vi "vizuXY_svi.vi"(9 "LY (mm)":dbl, 10 "LX (mm)":dbl, 11 "stored XY (µm)":T1 caption="stored XY") -> (3 "Tableau":T2(array[cluster]))   [LabVIEW 2013]
uses:
  <vilib>/Analysis/Matrix/Datatypes/RealMatrix.ctl
  <vilib>/Analysis/Matrix/Numeric/Conversions/Matrix To Array - RM.vi
  <vilib>/Analysis/Matrix/NI_Matrix.lvlib
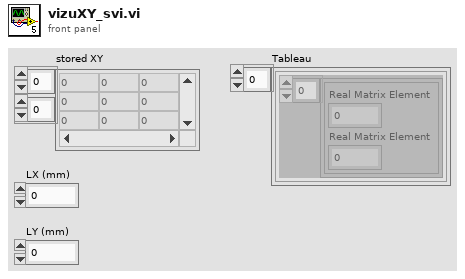
[diagram p1: front panel]
types:
  T1 = typedef "NI_Matrix.lvlib/RealMatrix.ctl" = dbl[][]
  T2 = cluster{cluster{"Real Matrix Element":dbl, "Real Matrix Element":dbl}[]}[]
  T3 = cluster{"Real Matrix Element":dbl, "Real Matrix Element":dbl}
  T4 = cluster{cluster{"Real Matrix Element":dbl, "Real Matrix Element":dbl}[]}
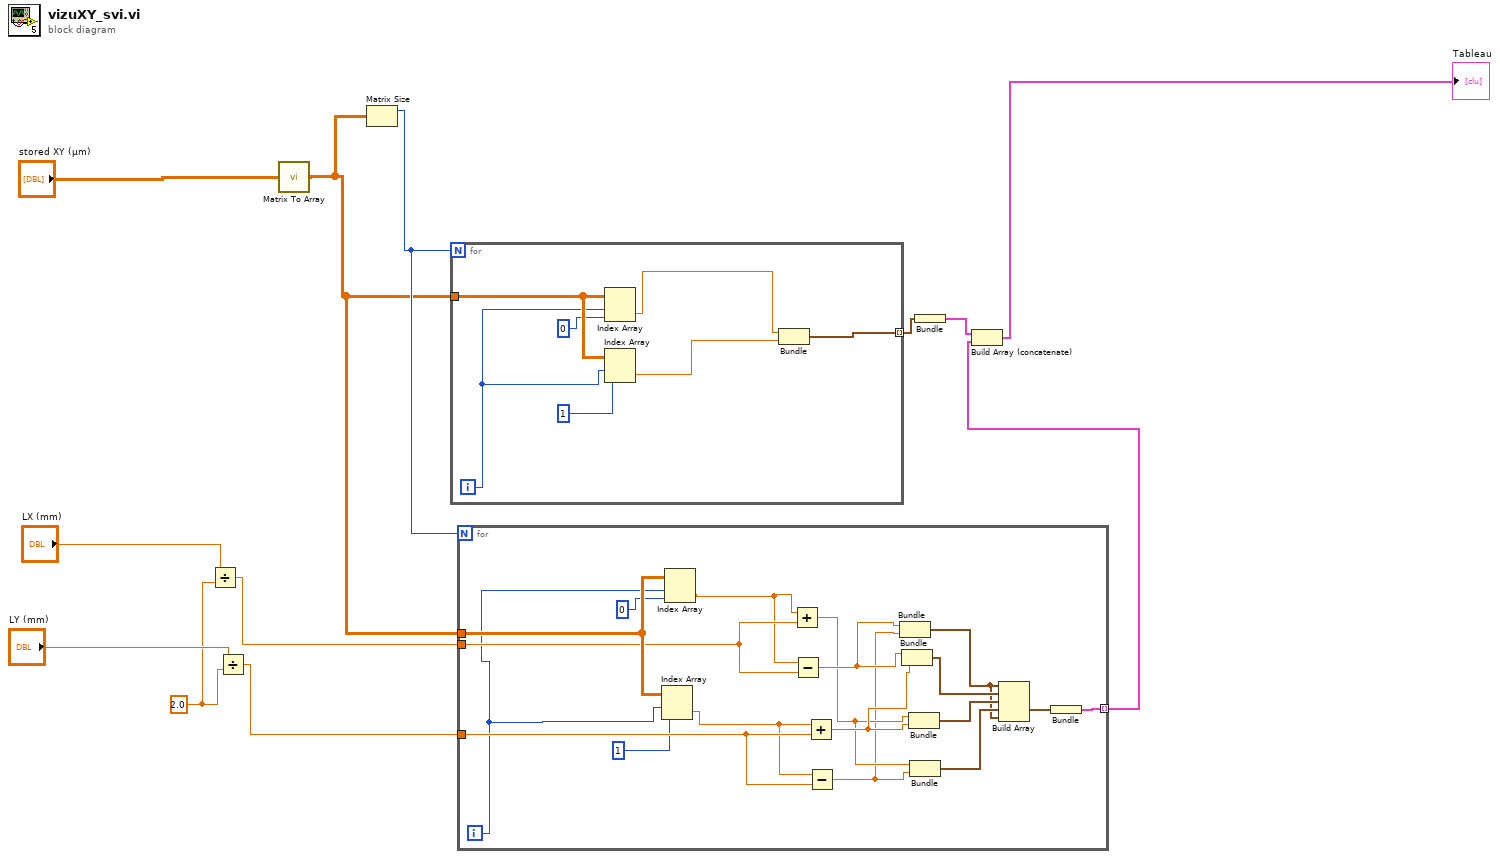
[diagram p0: block diagram]
diagram:
  w5 = 2.0
  n1 = Divide(x="LX (mm)", y=w5) -> (x/y=w6:dbl)
  n2 = Divide(x="LY (mm)", y=w5) -> (x/y=w7:dbl)
  n3 = call-poly <vilib>:"Matrix To Array.vi"("Real Matrix"="stored XY (µm)") -> ("Real 2D Array"=w4:dbl[][])
  n4 = Matrix Size(0:w4) -> (1:w9:i32)  [unwired: 1 out]
  n5 = for {
    N: w9 -> [_]
    tunnel: w4 -> [w19]
    tunnel: [w15] -> w2 mode=indexing
    i -> [w17]
    n6 = Index Array(array=w19, index (row)=w17, index (col)=0) -> (element=w13:dbl)
    n7 = Index Array(array=w19, index (row)=w17, index (col)=1) -> (element=w14:dbl)
    n8 = Bundle("Real Matrix Element"=w13, "Real Matrix Element"=w14) -> (w15:T3)  [unwired: 1 in]
  }
  n9 = for {
    N: w9 -> [_]
    tunnel: w4 -> [w37]
    tunnel: w6 -> [w36]
    tunnel: w7 -> [w35]
    tunnel: [w34] -> w10 mode=indexing
    i -> [w22]
    n10 = Index Array(array=w37, index (row)=w22, index (col)=1) -> (element=w21:dbl)
    n11 = Index Array(array=w37, index (row)=w22, index (col)=0) -> (element=w20:dbl)
    n12 = Add(x=w20, y=w36) -> (x+y=w29:dbl)
    n13 = Subtract(x=w20, y=w36) -> (x-y=w31:dbl)
    n14 = Add(x=w21, y=w35) -> (x+y=w30:dbl)
    n15 = Subtract(x=w21, y=w35) -> (x-y=w28:dbl)
    n16 = Bundle(w31, w28) -> (w23:cluster{dbl, dbl})  [unwired: 1 in]
    n17 = Bundle(w31, w30) -> (w27:cluster{dbl, dbl})  [unwired: 1 in]
    n18 = Bundle(w29, w30) -> (w26:cluster{dbl, dbl})  [unwired: 1 in]
    n19 = Bundle(w29, w28) -> (w25:cluster{dbl, dbl})  [unwired: 1 in]
    n20 = Build Array(w23, w27, w26, w25, w23) -> (w24:cluster{dbl, dbl}[])
    n21 = Bundle(w24) -> (w34:cluster{cluster{dbl, dbl}[]})  [unwired: 1 in]
  }
  n22 = Bundle(w2) -> (w3:T4)  [unwired: 1 in]
  n23 = Build Array (concatenate)(w3, w10) -> (→"Tableau":T2)
